vi "Read Lister Data.vi"(8 "error in (no error)":errorcluster, 9 "Display Window Type (0: Packets)":i32(ring) items=["Packets", "Symbols"], 10 "Serial Bus Number (0: Serial Bus 1)":i32(ring) items=["Serial Bus 1", "Serial Bus 2", "Serial Bus 3", "Serial Bus 4"], 11 "VISA resource name":refnum<visa-resource-name>) -> (0 "error out":errorcluster, 2 "Lister Data":string, 3 "VISA resource name out":refnum<visa-resource-name>)   [LabVIEW 2020, in "Agilent 90000 Series.lvlib"]
doc: "Queries the lister data."
uses:
  Agilent 90000 Series.lvlib
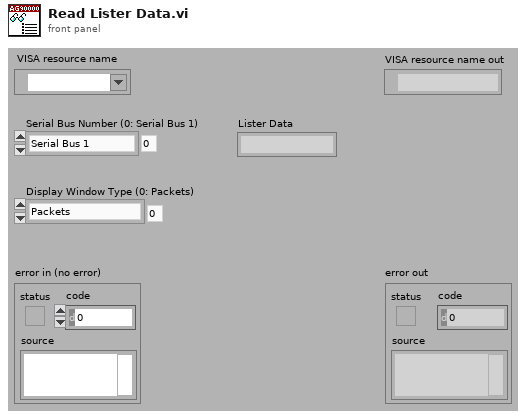
[diagram p1: front panel]
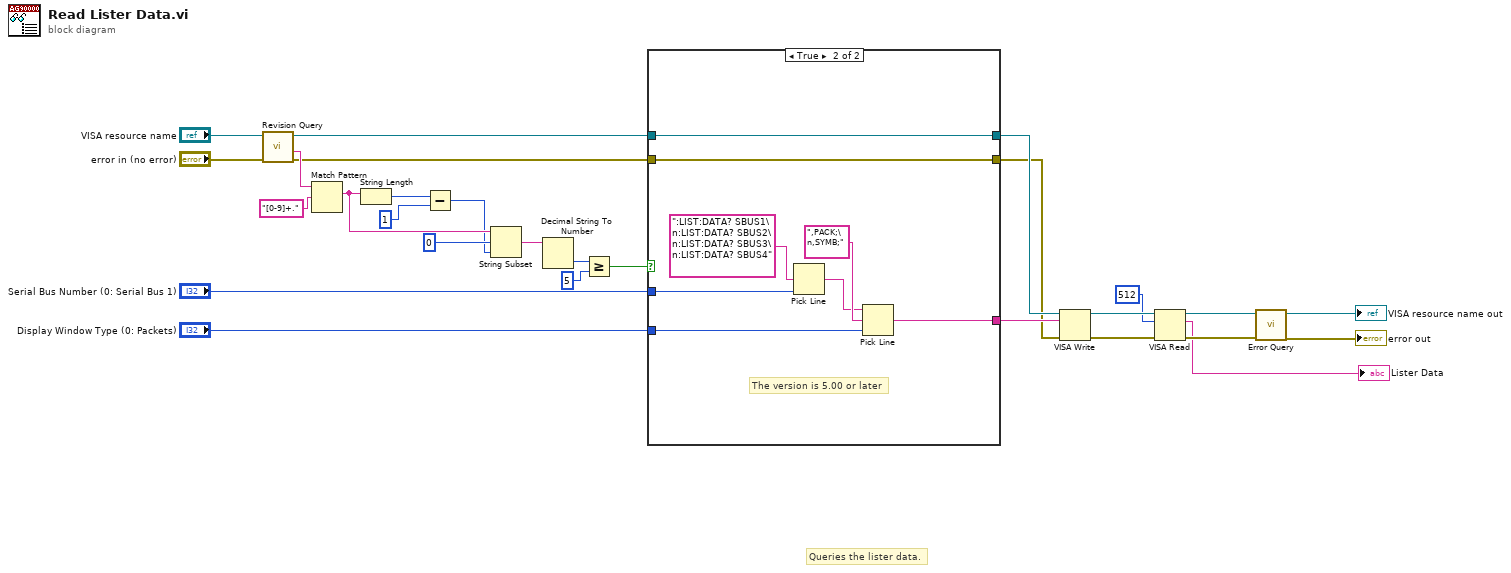
[diagram p0: block diagram]
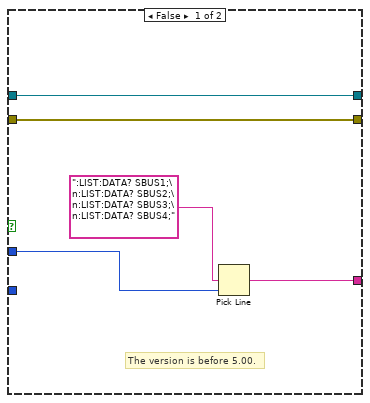
[diagram p2: hidden frame]
diagram:
  # "Queries the lister data."
  n1 = call "Revision Query.vi"("error in (no error)"="error in (no error)", "VISA resource name"="VISA resource name") -> ("error out"=w4:errorcluster, "Instrument Firmware Revision"=w11:string, "VISA resource name out"=w5:refnum<visa-resource-name>)  [unwired: 6 in, 1 out]
  n2 = Match Pattern(string=w11, regular expression="[0-9]+.") -> (match substring=w19:string)  [unwired: 1 in, 3 out]
  n3 = String Length(string=w19) -> (length=w17:i32)
  n4 = Subtract(x=w17, y=1) -> (x-y=w15:i32)
  n5 = String Subset(string=w19, offset (0)=0, length (rest)=w15) -> (substring=w14:string)
  n6 = Decimal String To Number(string=w14) -> (number=w13:i32)  [unwired: 2 in, 1 out]
  n7 = Greater Or Equal?(x=w13, y=5) -> (x >= y?=w8:bool)
  n8 = case shown="True" w8 {
    tunnel: "Serial Bus Number (0: Serial Bus 1)" -> [w32 w41]
    tunnel: [w31 w34] -> w6
    tunnel: w5 -> [w30 w40]
    tunnel: [w30 w40] -> w3
    tunnel: w4 -> [w29 w39]
    tunnel: [w29 w39] -> w2
    tunnel: "Display Window Type (0: Packets)" -> [_ w35]
    frame False {
      # "The version is before 5.00."
      n9 = Pick Line(multi-line string=":LIST:DATA? SBUS1;\n:LIST:DATA? SBUS2;\n:LIST:DATA? SBUS3;\n:LIST:DATA? SBUS4;", line index=w32) -> (output string=w31:string)  [unwired: 1 out]
    }
    frame True {
      # "The version is 5.00 or later"
      n10 = Pick Line(multi-line string=":LIST:DATA? SBUS1\n:LIST:DATA? SBUS2\n:LIST:DATA? SBUS3\n:LIST:DATA? SBUS4", line index=w41) -> (output string=w36:string)  [unwired: 1 out]
      n11 = Pick Line(string ("")=w36, multi-line string=",PACK;\n,SYMB;", line index=w35) -> (output string=w34:string)
    }
  }
  n12 = VISA Write(VISA resource name=w3, write buffer=w6, error in (no error)=w2) -> (VISA resource name out=w26:refnum<visa-resource-name>, error out=w25:errorcluster)  [unwired: 1 out]
  n13 = VISA Read(VISA resource name=w26, byte count=u32 512, error in (no error)=w25) -> (VISA resource name out=w24:refnum<visa-resource-name>, read buffer=→"Lister Data":string, error out=w23:errorcluster)  [unwired: 1 out]
  n14 = call "Error Query.vi"("error in (no error)"=w23, "VISA resource name"=w24) -> ("error out"=→"error out":errorcluster, "VISA resource name out"=→"VISA resource name out":refnum<visa-resource-name>)  [unwired: 8 out]
